vi "Read Outputs.vi"(8 "error in (no error)":errorcluster, 11 "LogicIO in":refnum<class "LogicIO.lvclass">) -> (0 "error out":errorcluster, 2 "LogicOutputs":bool[](array[boolean]), 3 "LogicIO out":refnum<class "LogicIO.lvclass">)   [LabVIEW 2016, in "Hardware.lvlib" / "LogicIO.lvlib" / "LogicIO.lvclass"]
uses:
  <userlib>/Common Components/Hardware/LogicIO/LogicIO/LogicIO.lvclass
panel:
  # "Outputs are sent to the notifier"
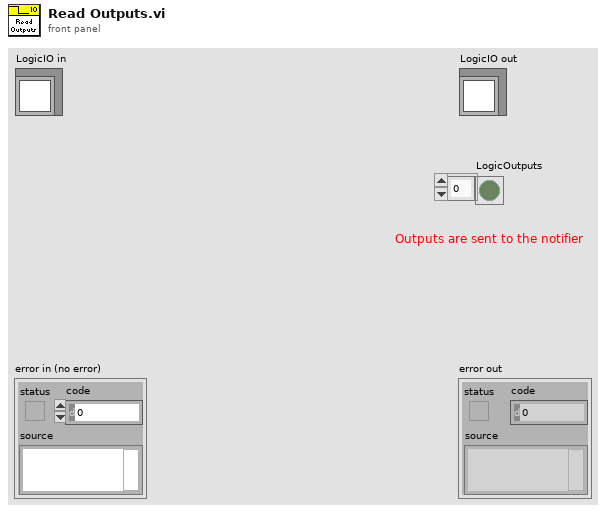
[diagram p1: front panel]
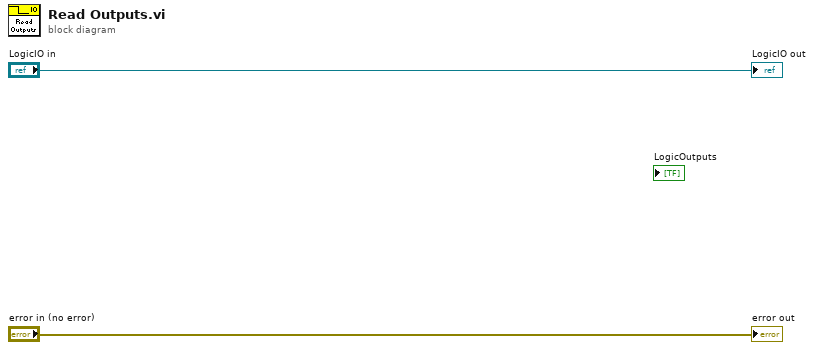
[diagram p0: block diagram]
diagram:
  "error out" <- "error in (no error)"
  "LogicIO out" <- "LogicIO in"
